vi "MainPHUdemo.vi"() -> ()   [LabVIEW 2020]
doc: "Read Binary File opens and reads an existing file stored as a double precision array in binary form. This VI shows the simplest way to read this entire file, with the simplest error checking."
panel:
  out "Histogram":u32[][](graph)
  out "Histograms":u32[][](array[numeric])
  out "HistoBinWidth":dbl[](array[numeric])
  out "NumOfHistoBins":i64[](array[numeric])
  out "NumberOfCurves":i64 format="%x"
  out "n_hdr_items":i32=80
  out "Version":string
  out "Magic":string
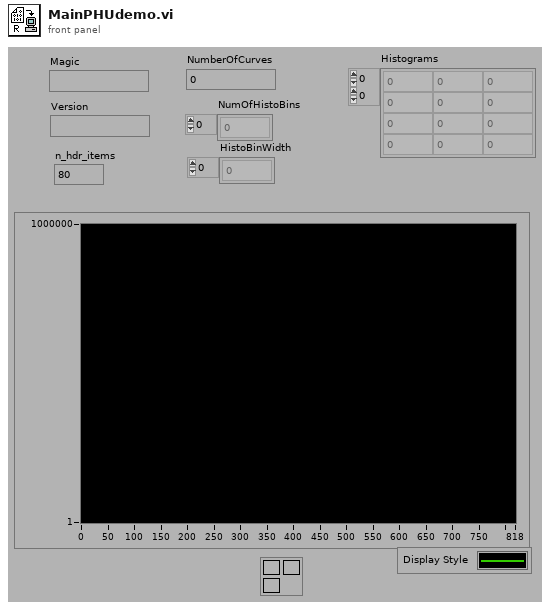
[diagram p1: front panel]
types:
  T1 = cluster{"TagIdent":string, "TagIndex":i32, "TagType":i32, "TagValue":i64, "TagAuxData":string}
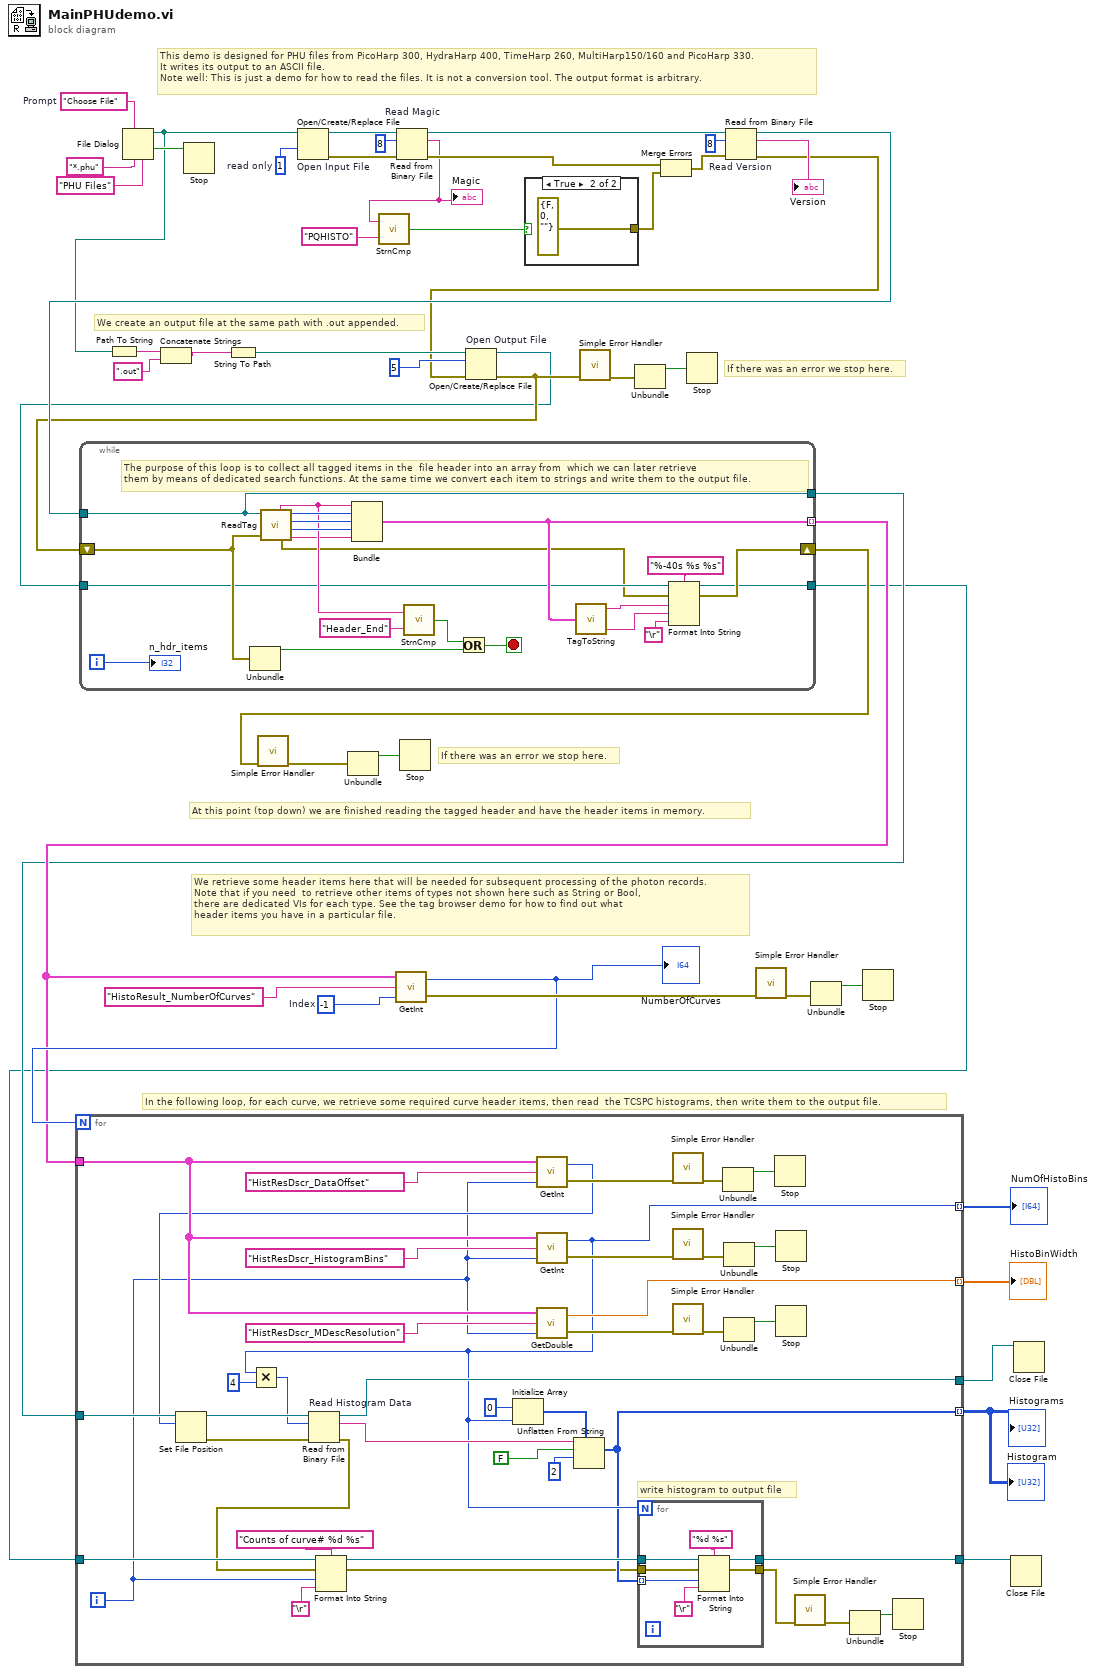
[diagram p0: block diagram]
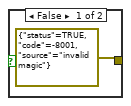
[diagram p2: hidden frame]
diagram:
  w28 = -1  # Index
  w1 = 1  # read only
  w46 = "Choose File"  # Prompt
  # "This demo is designed for PHU files from PicoHarp 300, HydraHarp 400, TimeHarp 260, MultiHarp150/160 and PicoHarp 330. \nIt writes its output to an ASCII file.\nNote well: This is just a demo for how to read the files. It is not a conversion tool. The output format is arbitrary."
  # "In the following loop, for each curve, we retrieve some required curve header items, then read  the TCSPC histograms, then write them to the output file."
  # "If there was an error we stop here."
  # "We create an output file at the same path with .out appended."
  # "If there was an error we stop here."
  # "At this point (top down) we are finished reading the tagged header and have the header items in memory."
  # "We retrieve some header items here that will be needed for subsequent processing of the photon records.\nNote that if you need  to retrieve other items of types not shown here such as String or Bool, \nthere are dedicated VIs for each type. See the tag browser demo for how to find out what \nheader items you have in a particular file."
  n1 = File Dialog(4:"PHU Files", 6:"*.phu", 7:w46) -> (1:w32:bool, 3:w23:path)  [unwired: 4 in, 2 out]
  n2 = Path To String(path=w23) -> (string=w22:string)
  n3 = Concatenate Strings(w22, ".out" ("string")) -> (w20:string)
  n4 = Stop(stop? (T)=w32) -> ()
  n5 = String To Path(string=w20) -> (path=w19:path)
  n6 = Open/Create/Replace File "Open Input File"(file path (use dialog)=w23, access (0:read/write)=w1) -> (refnum out=w34:refnum<file>, error out=w33:errorcluster)  [unwired: 4 in, 1 out]
  n7 = Read from Binary File "Read Magic"(8:w33, 10:8, 11:w34) -> (0:w41:errorcluster, 2:w37:string, 3:w45:refnum<file>)  [unwired: 3 in, 1 out]
  "Magic" <- w37
  n8 = call "StrnCmp.vi"("String 2"="PQHISTO", "String 1"=w37) -> ("equal"=w38:bool)
  n9 = case shown="True" w38 {
    tunnel: [errorcluster {"status"=TRUE, "code"=-8001, "source"="invalid magic"} ("file error status 2") errorcluster {"status"=FALSE, "code"=0, "source"=""} ("file error status 2")] -> w39
    frame False {
    }
    frame True {
    }
  }
  n10 = Merge Errors(w41, w39) -> (w40:errorcluster)
  n11 = Read from Binary File "Read Version"(8:w40, 10:8, 11:w45) -> (0:w16:errorcluster, 2:→"Version":string, 3:w31:refnum<file>)  [unwired: 3 in, 1 out]
  n12 = Open/Create/Replace File "Open Output File"(file path (use dialog)=w19, error in=w16, operation (0:open)=5) -> (refnum out=w13:refnum<file>, error out=w15:errorcluster)  [unwired: 3 in, 1 out]
  n13 = while {
    shift-left: w15 -> [w68]
    shift-right: [w54] -> w26
    tunnel: w31 -> [w50]
    tunnel: [w58] -> w11 mode=indexing
    tunnel: w13 -> [w57]
    tunnel: [w51] -> w5
    tunnel: [w50] -> w8
    i -> [w64]
    stop <- w69 stop-if-true
    # "The purpose of this loop is to collect all tagged items in the  file header into an array from  which we can later retrieve \nthem by means of dedicated search functions. At the same time we convert each item to strings and write them to the output file."
    n14 = Unbundle(w68) -> ("status"=w61:bool)  [unwired: 2 out]
    n15 = call "ReadTag.vi"("refnum"=w50, "error in"=w68) -> ("TagIdent"=w60:string, "TagIndex"=w67:i32, "TagType"=w66:i32, "error out"=w55:errorcluster, "TagValue"=w65:i64, "TagAuxData"=w59:string)  [unwired: 3 in]
    n16 = Bundle("TagIdent"=w60, "TagIndex"=w67, "TagType"=w66, "TagValue"=w65, "TagAuxData"=w59) -> (w58:T1)  [unwired: 1 in]
    n17 = call "StrnCmp.vi"("String 2"="Header_End", "String 1"=w60) -> ("equal"=w62:bool)
    n18 = Or(x=w62, y=w61) -> (x .or. y?=w69:bool)
    n19 = call "TagToString.vi"("TagData"=w58) -> ("StrTagValue"=w52:string, "StrTagName"=w53:string)  [unwired: 2 in, 1 out]
    n20 = Format Into String(format string="%-40s %s %s", initial string=w57, error in=w55, w53, w52, "\r") -> (resulting string=w51:refnum<file>, error out=w54:errorcluster)
    "n_hdr_items" <- w64
  }
  n21 = call <vilib>:"Simple Error Handler.vi"("error in (no error)"=w26) -> ("error out"=w25:errorcluster)  [unwired: 4 in, 4 out]
  n22 = Unbundle(w25) -> ("status"=w24:bool)  [unwired: 2 out]
  n23 = call "GetInt.vi"("Index"=w28, "Ident"="HistoResult_NumberOfCurves", "Array"=w11) -> ("error status"=w27:errorcluster, "TagValue"=w12:i64)
  "NumberOfCurves" <- w12
  n24 = for {
    N: w12 -> [_]
    tunnel: w11 -> [w102]
    tunnel: [w89] -> w10 mode=indexing
    tunnel: [w101] -> w9 mode=indexing
    tunnel: w8 -> [w100]
    tunnel: [w97] -> w7
    tunnel: [w82] -> w6 mode=indexing
    tunnel: w5 -> [w87]
    tunnel: [w83] -> w4
    i -> [w86]
    # "write histogram to output file"
    n25 = call "GetInt.vi"("Index"=w86, "Ident"="HistResDscr_DataOffset", "Array"=w102) -> ("error status"=w107:errorcluster, "TagValue"=w99:i64)
    n26 = Set File Position(offset (in bytes) (0)=w99, refnum=w100) -> (refnum out=w98:refnum<file>, error out=w77:errorcluster)  [unwired: 2 in]
    n27 = call "GetInt.vi"("Index"=w86, "Ident"="HistResDscr_HistogramBins", "Array"=w102) -> ("error status"=w105:errorcluster, "TagValue"=w89:i64)
    n28 = Multiply(x=w89, y=i64 4) -> (x*y=w95:i64)
    n29 = Read from Binary File "Read Histogram Data"(8:w77, 10:w95, 11:w98) -> (0:w76:errorcluster, 2:w90:string, 3:w97:refnum<file>)  [unwired: 3 in, 1 out]
    n30 = Format Into String(format string="Counts of curve# %d %s", initial string=w87, error in=w76, w86, "\r") -> (resulting string=w84:refnum<file>, error out=w81:errorcluster)
    n31 = Initialize Array(u32 0, w89) -> (w91:u32[])
    n32 = call "GetDouble.vi"("Index"=w86, "Ident"="HistResDscr_MDescResolution", "Array"=w102) -> ("error status"=w103:errorcluster, "TagValue"=w101:dbl)
    n33 = Unflatten From String(type=w91, binary string=w90, data includes array or string size? (T)=FALSE, byte order (0:big-endian, network order)=2) -> (value=w82:u32[])  [unwired: 1 in, 2 out]
    n34 = for {
      N: w89 -> [_]
      tunnel: w84 -> [w113]
      tunnel: [w112] -> w83
      tunnel: w82 -> [w111] mode=indexing
      tunnel: w81 -> [w110]
      tunnel: [w109] -> w79
      n35 = Format Into String(format string="%d %s", initial string=w113, error in=w110, w111, "\r") -> (resulting string=w112:refnum<file>, error out=w109:errorcluster)
    }
    n36 = call <vilib>:"Simple Error Handler.vi"("error in (no error)"=w107) -> ("error out"=w72:errorcluster)  [unwired: 4 in, 4 out]
    n37 = call <vilib>:"Simple Error Handler.vi"("error in (no error)"=w105) -> ("error out"=w71:errorcluster)  [unwired: 4 in, 4 out]
    n38 = call <vilib>:"Simple Error Handler.vi"("error in (no error)"=w103) -> ("error out"=w70:errorcluster)  [unwired: 4 in, 4 out]
    n39 = Unbundle(w72) -> ("status"=w75:bool)  [unwired: 2 out]
    n40 = Unbundle(w71) -> ("status"=w74:bool)  [unwired: 2 out]
    n41 = Unbundle(w70) -> ("status"=w73:bool)  [unwired: 2 out]
    n42 = Stop(stop? (T)=w75) -> ()
    n43 = Stop(stop? (T)=w74) -> ()
    n44 = Stop(stop? (T)=w73) -> ()
    n45 = call <vilib>:"Simple Error Handler.vi"("error in (no error)"=w79) -> ("error out"=w78:errorcluster)  [unwired: 4 in, 4 out]
    n46 = Unbundle(w78) -> ("status"=w80:bool)  [unwired: 2 out]
    n47 = Stop(stop? (T)=w80) -> ()
  }
  "NumOfHistoBins" <- w10
  "HistoBinWidth" <- w9
  "Histograms" <- w6
  "Histogram" <- w6
  n48 = Stop(stop? (T)=w24) -> ()
  n49 = call <vilib>:"Simple Error Handler.vi"("error in (no error)"=w15) -> ("error out"=w14:errorcluster)  [unwired: 4 in, 4 out]
  n50 = Unbundle(w14) -> ("status"=w17:bool)  [unwired: 2 out]
  n51 = Stop(stop? (T)=w17) -> ()
  n52 = call <vilib>:"Simple Error Handler.vi"("error in (no error)"=w27) -> ("error out"=w2:errorcluster)  [unwired: 4 in, 4 out]
  n53 = Unbundle(w2) -> ("status"=w3:bool)  [unwired: 2 out]
  n54 = Stop(stop? (T)=w3) -> ()
  n55 = Close File(refnum=w4) -> ()  [unwired: 1 in, 2 out]
  n56 = Close File(refnum=w7) -> ()  [unwired: 1 in, 2 out]
